vi "適應性控制_多頻率追蹤_V3(實際控制).vi"() -> ()   [LabVIEW 2010]
panel:
  in  "input Kp":dbl=1.0
  in  "理想初始頻率(Hz)":dbl=1.0
  in  "理想頻率數":i32=2
  out "當下誤差":dbl=0.1 format="%#_13g"
  out "實際輸入x(t)":dbl[][](graph)
  in  "頻率間距":dbl=1.0
  out "理想與FIR輸出":dbl[][](graph)
  out "message":string=" INSTRUCTIONS:\r\rNormal Use:  When using subVIs that incorporate the error in/error out (or error I/O) structure, place this handler where you want to inform the user of an error, typically at the end of the I/O data path, as the last action of the program.  If the error in error? is ERROR, the handler creates a message describing the error and its source.  If the type of dialog = 1 (default), the message is displayed to the user, who can only acknowedge it.  If the type = 2, the user can acknowledge the message or abort execution; aborting a program with active I/O is not recommended.  If the type = 0, no message is displayed; this is used to process the error programmatically, and the error out cluster elements are wired to individual terminals for that reason.  \r\rOther Use:\n\r\nlocal testing.  To test the error code of a subVI or function that does not have the error I/O structure, you can wire its error code and a source string to the local error code and error source inputs.  If error in error? indicates no error and error code is not equal to 0, the local code and source are substituted for the error in values, and error? is set TRUE (ERROR)."
  out "誤差":dbl(graph)
  out "while平均運行時間":dbl
  out "收斂time":dbl
  out "各頻率誤差已達標準":bool
  in  "各頻率誤差低於多少亮燈":dbl=0.1 format="%#_13g"
  out "權重(w)":dbl[](array[numeric])
  in  "理想振幅":dbl=0.5
  in  "理想直流偏移":dbl
  in  "理想相位(deg)":dbl
  in  "收斂係數":dbl=0.0001
  in  "order":i32=150
  in  "取樣頻率":dbl=150.0 min=1.0 max=10000.0 step=1.0
  in  "stop":bool
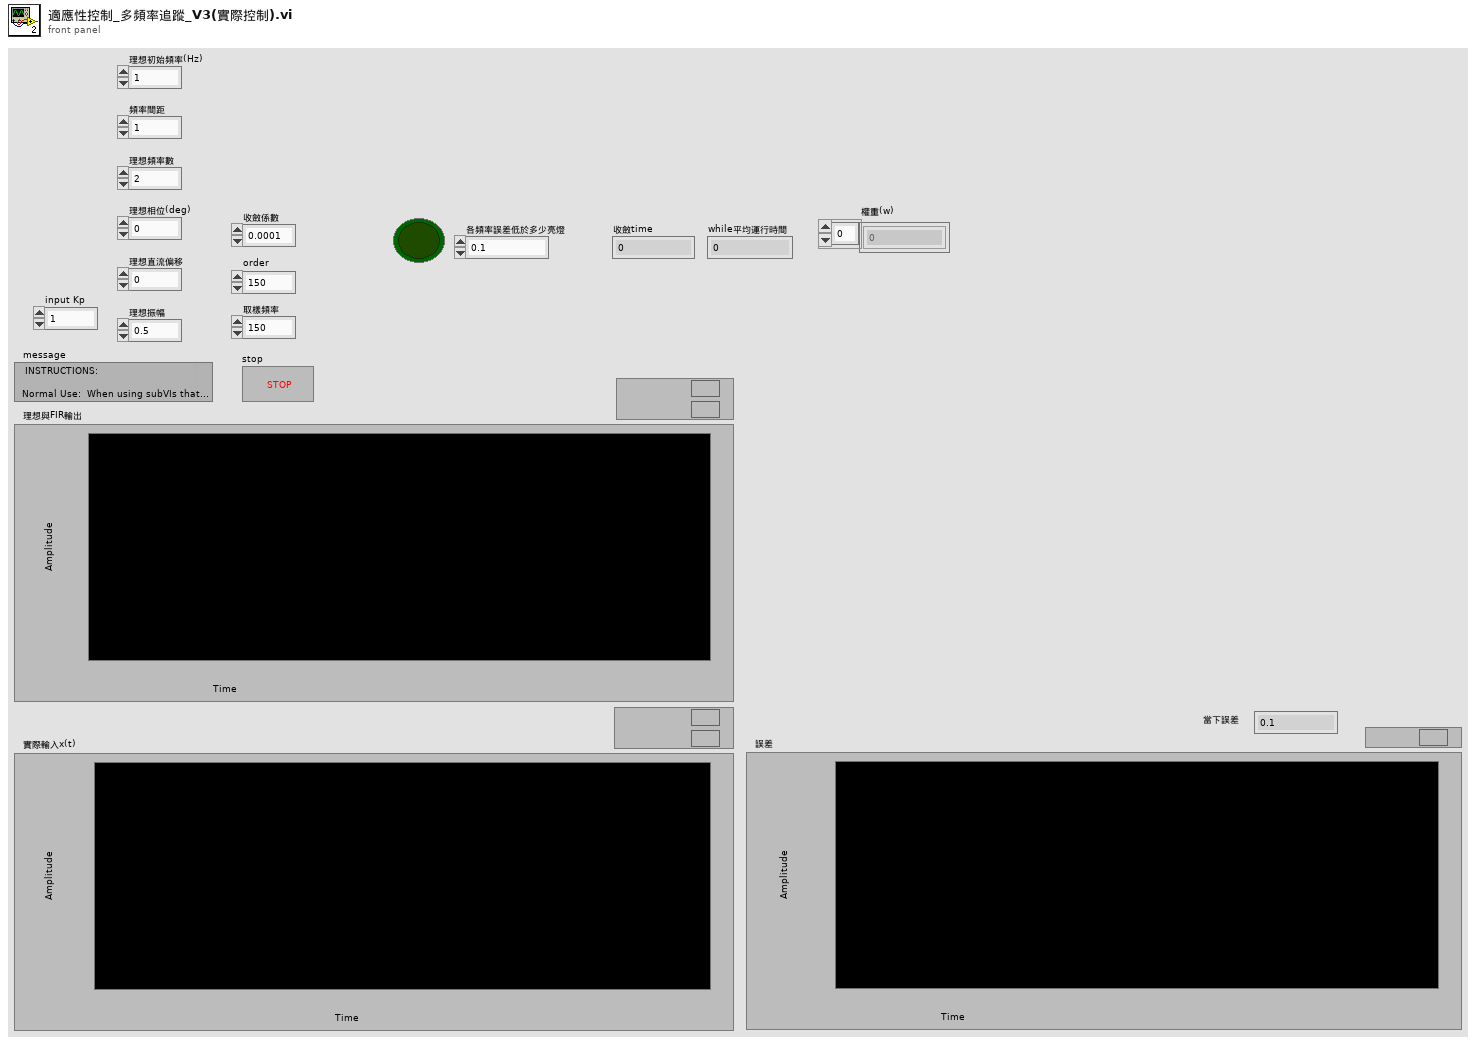
[diagram p1: front panel]
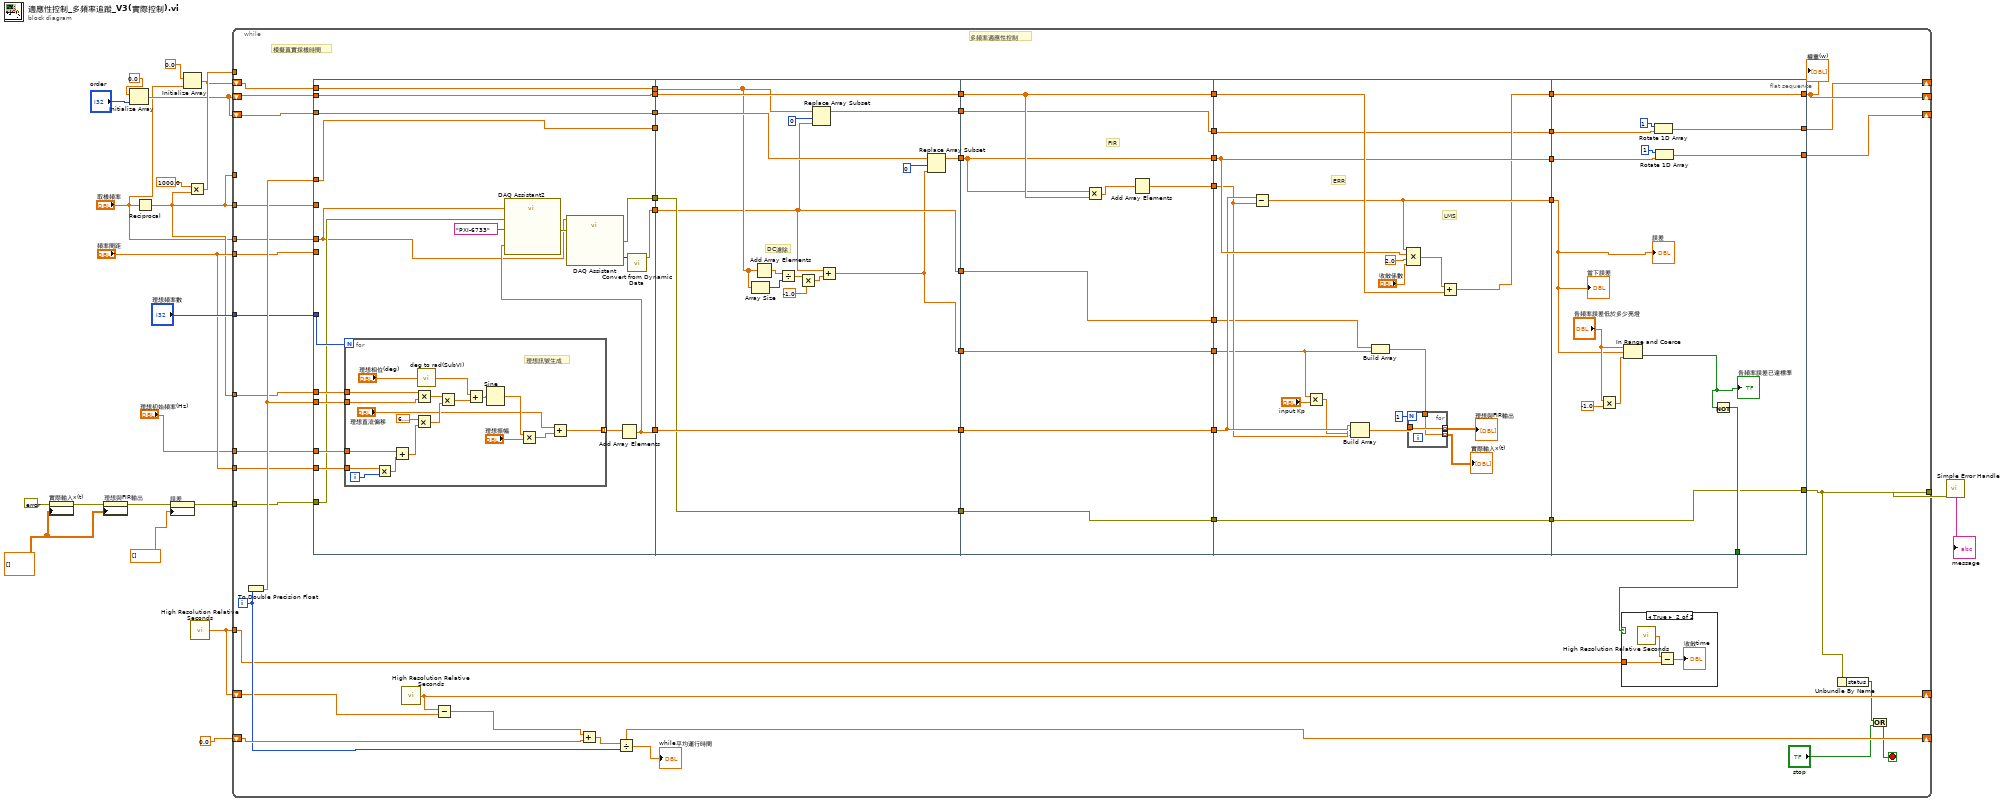
[diagram p0: block diagram]
diagram:
  w5 = dbl[][] [] ("History Data")
  n1 = property on="實際輸入x(t)" class="WFChart (strict)"(error in=errorcluster {"status"=FALSE, "code"=0, "source"=""} ("error constant"), "History Data"=w5) -> (error out=w13:errorcluster)  [unwired: 1 in, 1 out]
  n2 = property on="理想與FIR輸出" class="WFChart (strict)"(error in=w13, "History Data"=w5) -> (error out=w14:errorcluster)  [unwired: 1 in, 1 out]
  n3 = Initialize Array(0.0 ("element"), "order") -> (w4:dbl[])
  n4 = Reciprocal(x="取樣頻率") -> (1/x=w8:dbl)
  n5 = property on="誤差" class="WFChart (strict)"(error in=w14, "History Data"=dbl[] []) -> (error out=w16:errorcluster)  [unwired: 1 in, 1 out]
  n6 = Initialize Array(0.0 ("element"), "取樣頻率") -> (w3:dbl[])
  n7 = Multiply(x=1000.0, y=w8) -> (x*y=w20:dbl)
  n8 = call <vilib>:"High Resolution Relative Seconds.vi"() -> ("relative seconds"=w19:dbl)
  n9 = while {
    shift-right: [w42] -> _
    shift-left: w4 -> [w76]
    shift-right: [w63] -> _
    shift-left: w4 -> [w71]
    tunnel: w8 -> [_]
    tunnel: w8 -> [w60]
    tunnel: w20 -> [_]
    tunnel: w19 -> [w52]
    shift-right: [w53] -> _
    shift-left: w19 -> [w51]
    shift-right: [w54] -> _
    shift-left: 0.0 -> [w56]
    tunnel: [w26] -> w17
    tunnel: w16 -> [w46]
    tunnel: "頻率間距" -> [w45]
    tunnel: "理想頻率數" -> [w41]
    tunnel: "頻率間距" -> [w40]
    tunnel: "理想初始頻率(Hz)" -> [w39]
    tunnel: "取樣頻率" -> [w37]
    tunnel: w8 -> [w36]
    shift-right: [w30] -> _
    shift-left: w3 -> [w32]
    i -> [w55]
    stop <- w23 stop-if-true
    # "模擬真實採樣時間"
    # "多頻率適應性控制"
    n10 = To Double Precision Float(number=w55) -> (double precision float=w69:dbl)
    n11 = flat-sequence {
      tunnel: w69 -> [w82]
      tunnel: [w84] -> w77
      tunnel: w76 -> [w84]
      tunnel: [w85] -> w75
      tunnel: [w98] -> w72
      tunnel: w71 -> [w98]
      tunnel: w69 -> [w97]
      tunnel: [w89] -> w66
      tunnel: w60 -> [w96]
      tunnel: w46 -> [w91]
      tunnel: w45 -> [_]
      tunnel: w41 -> [w95]
      tunnel: w40 -> [w94]
      tunnel: w39 -> [w93]
      tunnel: [w87] -> w38
      tunnel: w37 -> [w83]
      tunnel: w36 -> [_]
      tunnel: [w82] -> w35
      tunnel: w32 -> [w81]
      tunnel: [w81] -> w31
      tunnel: w77 -> [w126]
      tunnel: w75 -> [w119]
      tunnel: [w133] -> w74
      tunnel: [w127] -> w73
      tunnel: w72 -> [w127]
      tunnel: [w132] -> w67
      tunnel: w66 -> [w132]
      tunnel: [w130] -> w47
      tunnel: [w119] -> w43
      tunnel: w38 -> [w130]
      tunnel: w35 -> [_]
      tunnel: [w118] -> w34
      tunnel: w31 -> [w123]
      tunnel: [w128] -> w27
      tunnel: w74 -> [w136]
      tunnel: w73 -> [w142]
      tunnel: [w142] -> w70
      tunnel: [w141] -> w68
      tunnel: w67 -> [w141]
      tunnel: [w140] -> w65
      tunnel: [w136] -> w64
      tunnel: [w139] -> w48
      tunnel: w47 -> [w139]
      tunnel: [w138] -> w44
      tunnel: w43 -> [w138]
      tunnel: w34 -> [w135]
      tunnel: [w135] -> w33
      tunnel: [w134] -> w29
      tunnel: w27 -> [w134]
      tunnel: w70 -> [w162]
      tunnel: w68 -> [w150]
      tunnel: w65 -> [w149]
      tunnel: w64 -> [w154]
      tunnel: [w151] -> w62
      tunnel: [w154] -> w61
      tunnel: [w155] -> w59
      tunnel: [w159] -> w49
      tunnel: w48 -> [w159]
      tunnel: w44 -> [w148]
      tunnel: w33 -> [w145]
      tunnel: w29 -> [w146]
      tunnel: [w146] -> w28
      tunnel: [w178] -> w63
      tunnel: w62 -> [w178]
      tunnel: w61 -> [w170]
      tunnel: [w177] -> w42
      tunnel: w59 -> [w168]
      tunnel: [w173] -> w50
      tunnel: [w172] -> w26
      tunnel: w49 -> [w172]
      tunnel: [w166] -> w30
      tunnel: w28 -> [w165]
      frame #0 {
        n12 = for {
          N: w95 -> [_]
          tunnel: w97 -> [w117]
          tunnel: [w116] -> w92 mode=indexing
          tunnel: w96 -> [w115]
          tunnel: w94 -> [w101]
          tunnel: w93 -> [w100]
          i -> [w102]
          # "理想訊號生成"
          n13 = Multiply(x=w101, y=w102) -> (x*y=w103:dbl)
          n14 = Add(x=w100, y=w103) -> (x+y=w99:dbl)
          n15 = Multiply(x=6.283185307179586, y=w99) -> (x*y=w112:dbl)
          n16 = Multiply(x=w115, y=w117) -> (x*y=w105:dbl)
          n17 = call "deg to rad(SubVI).vi"("Degree"="理想相位(deg)") -> ("Radian"=w109:dbl)
          n18 = Multiply(x=w105, y=w112) -> (x*y=w113:dbl)
          n19 = Add(x=w109, y=w113) -> (x+y=w114:dbl)
          n20 = Sine(x=w114) -> (sin(x)=w110:dbl)
          n21 = Multiply(x=w110, y="理想振幅") -> (x*y=w111:dbl)
          n22 = Add(x="理想直流偏移", y=w111) -> (x+y=w116:dbl)
        }
        n23 = Add Array Elements(numeric array=w92) -> (sum=w89:dbl)
        n24 = call "DAQ Assistant2"("data"=w89, "rate"=w83, "error in"=w91, "device name"=tag "PXI-6733") -> ("error out"=w88:errorcluster)  [unwired: 13 in, 2 out]
        n25 = call "DAQ Assistant"("rate"=w83, "error in"=w88) -> ("data"=w86:dynamicdata, "error out"=w87:errorcluster)  [unwired: 14 in, 2 out]
        n26 = call "Convert from Dynamic Data"("Dynamic Data Type"=w86) -> ("Scalar"=w85:dbl)  [unwired: 3 in]
      }
      frame #1 {
        # "DC濾除"
        n27 = Array Size(array=w123) -> (size(s)=w124:i32)
        n28 = Add Array Elements(numeric array=w123) -> (sum=w125:dbl)
        n29 = Divide(x=w125, y=w124) -> (x/y=w122:dbl)
        n30 = Multiply(x=w122, y=-1.0) -> (x*y=w120:dbl)
        n31 = Replace Array Subset(array=w123, new element=w119, index=0) -> (w128:dbl[])
        n32 = Add(x=w119, y=w120) -> (x+y=w118:dbl)
        n33 = Replace Array Subset(array=w126, new element=w118, index=0) -> (w133:dbl[])
      }
      frame #2 {
        # "FIR"
        n34 = Multiply(x=w136, y=w142) -> (x*y=w137:dbl[])
        n35 = Add Array Elements(numeric array=w137) -> (sum=w140:dbl)
      }
      frame #3 {
        # "LMS"
        # "ERR"
        n36 = Subtract(x=w150, y=w149) -> (x-y=w155:dbl)
        n37 = Multiply(x=w145, y="input Kp") -> (x*y=w143:dbl)
        n38 = Build Array(w150, w149, w143) -> (w160:dbl[])
        n39 = Build Array(w148, w145) -> (w147:dbl[])
        n40 = Compound Arithmetic op=MULTIPLY(w155, w154, 2.0, "收斂係數") -> (w153:dbl[])
        n41 = for {
          N: 1 -> [_]
          tunnel: [w164] -> w152 mode=indexing
          tunnel: w160 -> [w164]
          tunnel: [w163] -> w158 mode=indexing
          tunnel: w147 -> [w163]
        }
        "理想與FIR輸出" <- w152
        "實際輸入x(t)" <- w158
        n42 = Add(x=w153, y=w162) -> (x+y=w151:dbl[])
      }
      frame #4 {
        n43 = Multiply(x="各頻率誤差低於多少亮燈", y=-1.0) -> (x*y=w174:dbl)
        n44 = In Range and Coerce(upper limit="各頻率誤差低於多少亮燈", x=w168, lower limit=w174) -> (In Range?=w169:bool)  [unwired: 1 out]
        "各頻率誤差已達標準" <- w169
        n45 = Rotate 1D Array(1:w165, 2:1 ("n")) -> (0:w166:dbl[])
        n46 = Rotate 1D Array(1:w170, 2:1 ("n")) -> (0:w177:dbl[])
        n47 = Not(x=w169) -> (.not. x?=w173:bool)
        "誤差" <- w168
        "當下誤差" <- w168
      }
    }
    n48 = call <vilib>:"High Resolution Relative Seconds.vi"() -> ("relative seconds"=w53:dbl)
    n49 = Subtract(x=w53, y=w51) -> (x-y=w58:dbl)
    n50 = Add(x=w58, y=w56) -> (x+y=w54:dbl)
    n51 = Divide(x=w54, y=w55) -> (x/y=→"while平均運行時間":dbl)
    n52 = case shown="True" w50 {
      tunnel: w52 -> [_ w78]
      frame False {
      }
      frame True {
        n53 = call <vilib>:"High Resolution Relative Seconds.vi"() -> ("relative seconds"=w80:dbl)
        n54 = Subtract(x=w80, y=w78) -> (x-y=→"收斂time":dbl)
      }
    }
    n55 = Unbundle By Name(w26) -> ("status"=w25:bool)
    n56 = Or(x=w25, y="stop") -> (x .or. y?=w23:bool)
    "權重(w)" <- w63
  }
  n57 = call <vilib>:"Simple Error Handler.vi"("error in (no error)"=w17) -> ("message"=→"message":string)  [unwired: 4 in, 4 out]
